vi "Setup Red Pitaya.vi"() -> ()   [LabVIEW 2016]
panel:
  in  "Bitfiles to copy":path[](array[path])=[path "C:/github/fp/tmp/digitizer.bit", path "C:/github/fp/tmp/lockin_digitizer.bit", path "C:/github/fp/tmp/lockin_sweep.bit"]
  in  "Desired address":string="192.168.1.104"
  in  "Current address":string="192.168.1.100"
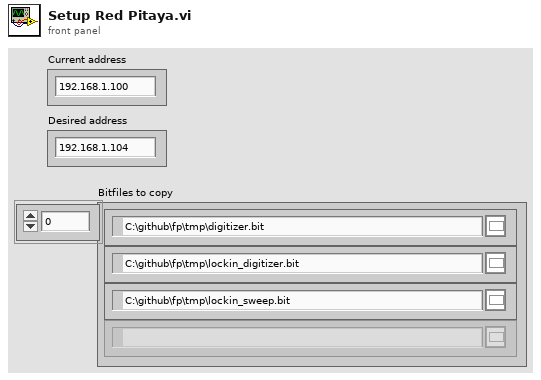
[diagram p1: front panel]
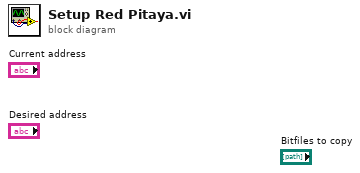
[diagram p0: block diagram]
diagram:
